vi "Read Spectral Waveform.vi"(8 "error in (no error)":errorcluster, 11 "VISA resource name":refnum<visa-resource-name>) -> (0 "error out":errorcluster, 2 "Spectral Waveform":cluster{dbl[], dbl[]}(graph), 3 "VISA resource name out":refnum<visa-resource-name>)   [LabVIEW 2013, in "Ocean Optics 2000 4000.lvlib"]
doc: "Displays the spectrum vs wavelength in a waveform graph.\n\n<b>Note:</b> Do not put this VI in a loop if performance is a concern. Please see the <b>Ocean Optics 2000 4000 Acquire Continuous Waveform</b> example for an example of how to do continuous acquisition."
uses:
  <instrlib>/Ocean Optics 2000 4000/Ocean Optics 2000 4000.lvlib
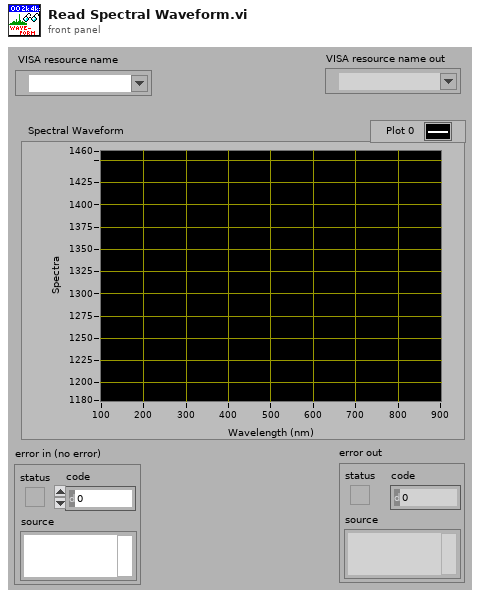
[diagram p1: front panel]
types:
  T1 = cluster{"Wavelength (nm)":dbl[], "Spectrum by Pixels":dbl[]}
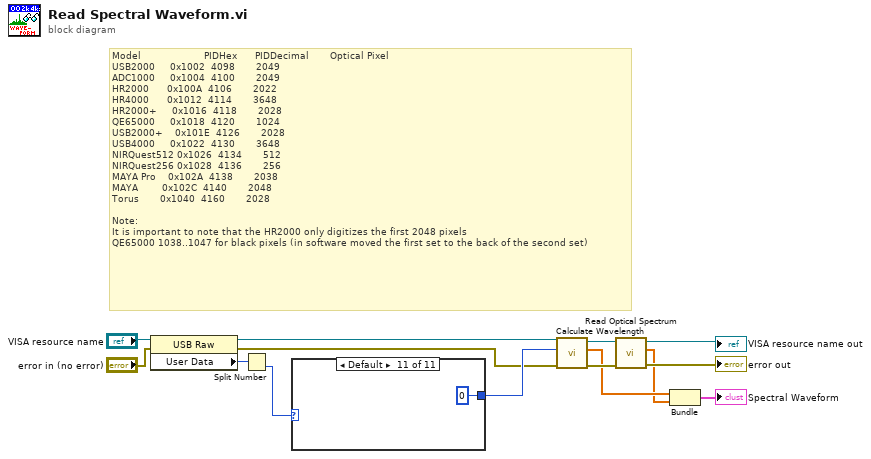
[diagram p0: block diagram]
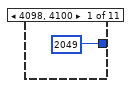
[diagram p2: hidden frame]
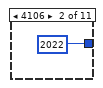
[diagram p3: hidden frame]
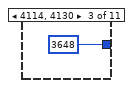
[diagram p4: hidden frame]
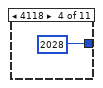
[diagram p5: hidden frame]
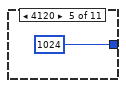
[diagram p6: hidden frame]
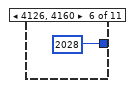
[diagram p7: hidden frame]
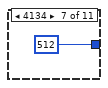
[diagram p8: hidden frame]
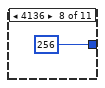
[diagram p9: hidden frame]
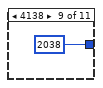
[diagram p10: hidden frame]
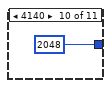
[diagram p11: hidden frame]
diagram:
  # "Model\t                    PIDHex     \tPIDDecimal      \tOptical Pixel\nUSB2000\t    0x1002\t 4098\t      2049\t\nADC1000\t    0x1004\t 4100\t      2049 \nHR2000\t     0x100A\t 4106\t      2022\t\nHR4000\t     0x1012\t 4114\t      3648\t\nHR2000+\t    0x1016\t 4118\t      2028\t\nQE65000\t    0x1018\t 4120\t      1024\t\nUSB2000+\t   0x101E\t 4126\t      2028\t\nUSB4000\t    0x1022\t 4130\t      3648\t\nNIRQuest512\t0x1026\t 4134\t      512\t \nNIRQuest256\t0x1028\t 4136\t      256\t \nMAYA Pro\t   0x102A\t 4138\t      2038\t\nMAYA\t       0x102C\t 4140\t      2048\t\nTorus\t      0x1040\t 4160\t      2028\t\n\nNote: \nIt is important to note that the HR2000 only digitizes the first 2048 pixels\nQE65000 1038..1047 for black pixels (in software moved the first set to the back of the second set)"
  n1 = property class="USB Raw"(reference="VISA resource name", error in="error in (no error)") -> (reference out=w2:refnum<visa-resource-name>, error out=w1:errorcluster, "User Data"=w5:u32)
  n2 = Split Number(x=w5) -> (lo(x)=w4:u16)  [unwired: 1 out]
  n3 = case shown="Default" w4 {
    tunnel: [2049 ("Number of Pixels (3840)") 2022 ("Number of Pixels (3840)") 3648 ("Number of Pixels (3840)") 2028 ("Number of Pixels (3840)") 1024 ("Number of Pixels (3840)") 2028 ("Number of Pixels (3840)") 512 ("Number of Pixels (3840)") 256 ("Number of Pixels (3840)") 2038 ("Number of Pixels (3840)") 2048 ("Number of Pixels (3840)") 0 ("Number of Pixels (3840)")] -> w3
    frame 4098, 4100 {
    }
    frame 4106 {
    }
    frame 4114, 4130 {
    }
    frame 4118 {
    }
    frame 4120 {
    }
    frame 4126, 4160 {
    }
    frame 4134 {
    }
    frame 4136 {
    }
    frame 4138 {
    }
    frame 4140 {
    }
    frame Default {
    }
  }
  n4 = call <instrlib>:"Calculate Wavelength.vi"("error in (no error)"=w1, "Number of Pixels (3648)"=w3, "VISA resource name"=w2) -> ("error out"=w10:errorcluster, "Wavelength (nm)"=w9:dbl[], "VISA resource name out"=w11:refnum<visa-resource-name>)  [unwired: 6 in]
  n5 = call <instrlib>:"Read Optical Spectrum.vi"("error in (no error)"=w10, "VISA resource name"=w11) -> ("error out"=→"error out":errorcluster, "Spectrum by Pixels"=w8:dbl[], "VISA resource name out"=→"VISA resource name out":refnum<visa-resource-name>)  [unwired: 6 in, 1 out]
  n6 = Bundle("Wavelength (nm)"=w9, "Spectrum by Pixels"=w8) -> (→"Spectral Waveform":T1)  [unwired: 1 in]
